vi "convertFromFPGA.vi"(0 "Modbus in":refnum<class "Modbus.lvclass">, 5 "Data":u16[](array[numeric]), 7 "StartIndex":i32, 9 "StopIndex":i32, 11 "error in (no error)":errorcluster) -> (4 "Modbus out":refnum<class "Modbus.lvclass">, 6 "Frame":T1={"Data"=[], "WaitForTrigger"=FALSE, "WaitForRx"=0, "TriggerIRQ"=-1} {"Data" format="%02x"}, 15 "error out":errorcluster)   [LabVIEW 2015, in "Modbus.lvclass"]
uses:
  Modbus.lvclass
  Typedefs/Frame.ctl
  Typedefs/RTTypeDefs.lvlib
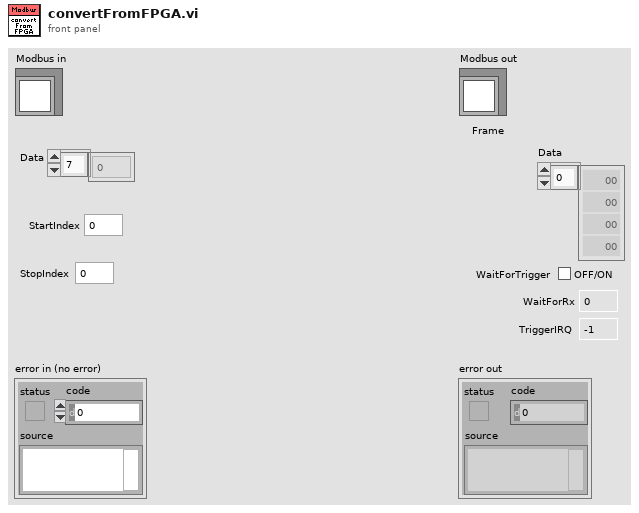
[diagram p1: front panel]
types:
  T1 = typedef "RTTypeDefs.lvlib/Frame.ctl" = cluster{"Data":u8[], "WaitForTrigger":bool, "WaitForRx":u16, "TriggerIRQ":i16}
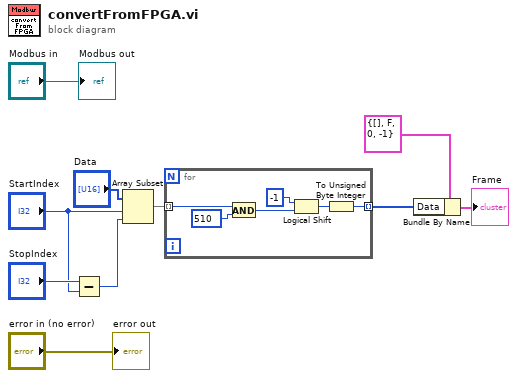
[diagram p0: block diagram]
diagram:
  n1 = Subtract(x="StopIndex", y="StartIndex") -> (x-y=w7:i32)
  n2 = Array Subset(array="Data", index="StartIndex", length=w7) -> (w6:u16[])
  n3 = for {
    tunnel: w6 -> [w11] mode=indexing
    tunnel: [w12] -> w1 mode=indexing
    n4 = And(x=w11, y=u16 510) -> (x .and. y?=w14:u16)
    n5 = Logical Shift(y=i16 -1, x=w14) -> (x << y=w13:u16)
    n6 = To Unsigned Byte Integer(number=w13) -> (unsigned 8bit integer=w12:u8)
  }
  n7 = Bundle By Name(cluster=T1 {"Data"=[], "WaitForTrigger"=FALSE, "WaitForRx"=0, "TriggerIRQ"=-1} ("Frame"), "Data"=w1) -> (→"Frame":T1)
  "error out" <- "error in (no error)"
  "Modbus out" <- "Modbus in"
